vi "Check Variant Type.vi"(8 "error in (no error)":errorcluster, 10 "Variant":variant, 11 "Timestamp Value in":refnum<class "Timestamp Value.lvclass">) -> (0 "error out":errorcluster, 3 "Timestamp Value out":refnum<class "Timestamp Value.lvclass">)   [LabVIEW 2020, in "Composed Columns.lvlib" / "Timestamp Value.lvclass"]
uses:
  Timestamp Value.lvclass
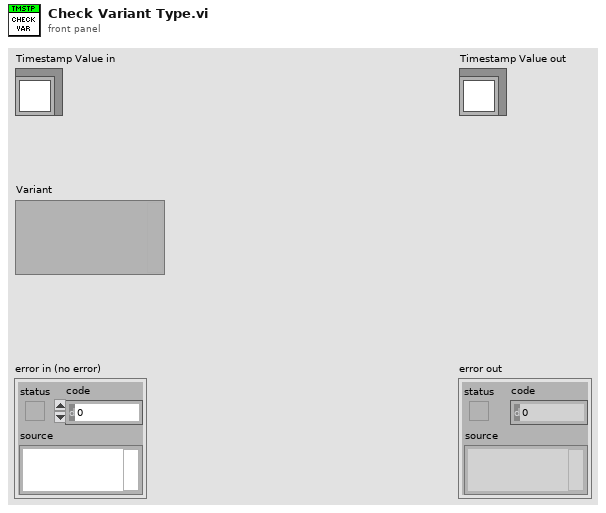
[diagram p1: front panel]
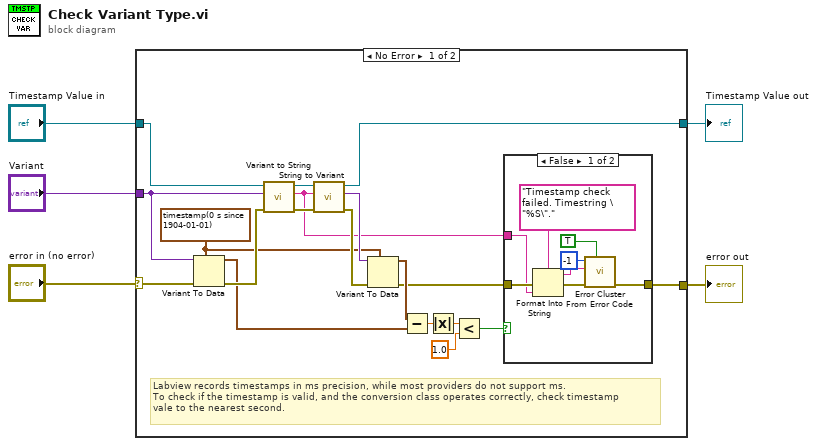
[diagram p0: block diagram]
diagram:
  n1 = case shown="No Error" "error in (no error)" {
    selector: "error in (no error)" -> [w21 w35]
    tunnel: "Variant" -> [w20 _]
    tunnel: "Timestamp Value in" -> [w23 w34]
    tunnel: [w22 w34] -> w2
    tunnel: [w9 w35] -> w1
    frame No Error {
      w15 = timestamp(0 s since 1904-01-01)
      # "Labview records timestamps in ms precision, while most providers do not support ms.\nTo check if the timestamp is valid, and the conversion class operates correctly, check timestamp\nvale to the nearest second."
      n2 = Variant To Data(error in=w21, type=w15, Variant=w20) -> (data=w12:timestamp, error out=w18:errorcluster)
      n3 = call-dynamic "Variant to String.vi"("error in (no error)"=w18, "Variant"=w20, "Timestamp Value in"=w23) -> ("error out"=w17:errorcluster, "String"=w8:string, "Timestamp Value out"=w24:refnum<class "Timestamp Value.lvclass">)  [unwired: 6 in]
      n4 = call-dynamic "String to Variant.vi"("error in (no error)"=w17, "String"=w8, "Timestamp Value in"=w24) -> ("error out"=w16:errorcluster, "Variant"=w19:variant, "Timestamp Value out"=w22:refnum<class "Timestamp Value.lvclass">)  [unwired: 6 in]
      n5 = Variant To Data(error in=w16, type=w15, Variant=w19) -> (data=w13:timestamp, error out=w10:errorcluster)
      n6 = Subtract(x=w13, y=w12) -> (x-y=w14:dbl)
      n7 = Absolute Value(x=w14) -> (abs(x)=w7:dbl)
      n8 = Less?(x=w7, y=1.0 ("x")) -> (x < y?=w11:bool)
      n9 = case shown="False" w11 {
        tunnel: w10 -> [w32 w33]
        tunnel: [w26 w33] -> w9
        tunnel: w8 -> [w25 _]
        frame False {
          n10 = Format Into String(format string="Timestamp check failed. Timestring \"%S\".", error in=w32, w25) -> (resulting string=w29:string, error out=w30:errorcluster)  [unwired: 1 in]
          n11 = call <vilib>:"Error Cluster From Error Code.vi"("show call chain? (False)"=TRUE, "error in (no error)"=w30, "error message (\"\")"=w29, "error code (0)"=-1) -> ("error out"=w26:errorcluster)  [unwired: 5 in]
        }
        frame True {
        }
      }
    }
    frame Error {
    }
  }
  "error out" <- w1
  "Timestamp Value out" <- w2
